vi "Init Panels.vi"(8 "error in (no error)":errorcluster, 11 "Editor in":refnum<class "Editor.lvclass">) -> (0 "error out":errorcluster, 3 "Editor out":refnum<class "Editor.lvclass">)   [LabVIEW 2020, in "VolatusGUIEditor.lvlib" / "Editor.lvclass"]
uses:
  Editor.lvclass
  Panels.ctl
  VolatusGUIControls/ElementEditorPanel/ElementEditorPanel.lvclass
  C:/dev/lv20CE/relink/lv-oopanel/OOPanel/Panel/Panel.lvclass
  ControlBindingPanel/ControlBindingPanel.lvclass
  Editor.lvclass/Editor.ctl
  lv-oopanel/OOPanel/Manager/Manager.lvclass
  Control List/Control List.lvclass
  VolatusGUIEditor.lvlib
  C:/dev/lv20CE/relink/volatus-gui-controls/VolatusGUIControls/ElementEditorPanel/ElementEditorPanel.lvclass
  C:/dev/lv20CE/relink/volatus-gui-controls/VolatusGUIEditor/ControlBindingPanel/ControlBindingPanel.lvclass
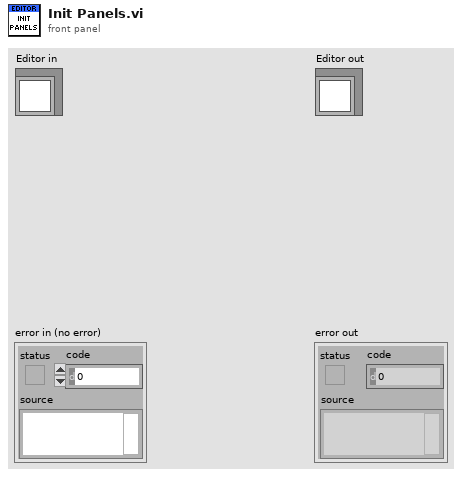
[diagram p1: front panel]
types:
  T1 = typedef "VolatusGUIEditor.lvlib/Editor.lvclass/Panels.ctl" = cluster{"Blank":refnum<class "ElementEditorPanel.lvclass">, "Binding":refnum<class "ControlBindingPanel.lvclass">}
  T2 = map{string, refnum<class "ElementEditorPanel.lvclass">}
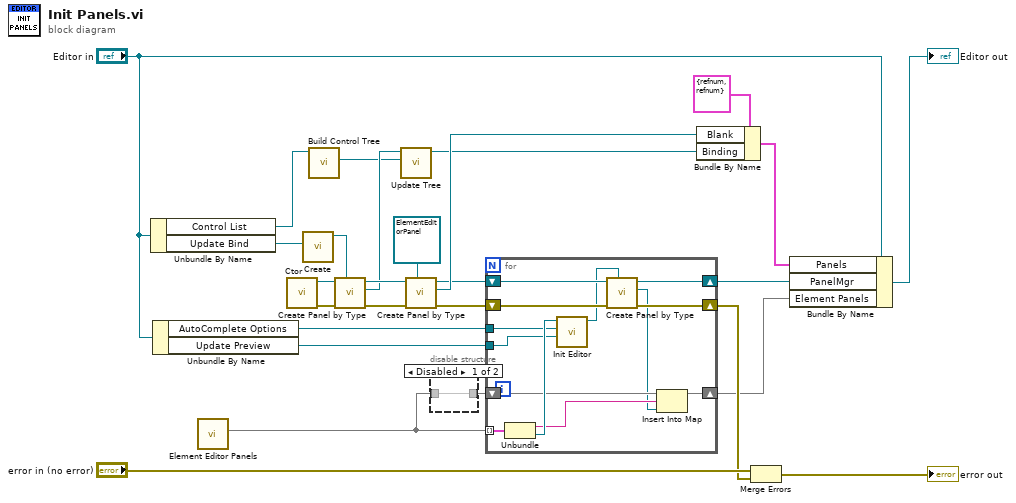
[diagram p0: block diagram]
diagram:
  n1 = Unbundle By Name("Editor in") -> ("Control List"=w12:refnum<class "Control List.lvclass">, "Update Bind"=w23:refnum<user-event>)
  n2 = Unbundle By Name("Editor in") -> ("AutoComplete Options"=w7:refnum<class "Shared Options.lvclass">, "Update Preview"=w3:refnum<user-event>)
  n3 = call "Element Editor Panels.vi"() -> ("Panels"=w5:T2)  [unwired: 11 in]
  n4 = call "Ctor.vi"() -> ("error out"=w25:errorcluster, "Manager out"=w26:refnum<class "Manager.lvclass">)  [unwired: 10 in]
  n5 = call "Create.vi"("Update Bind"=w23) -> ("ControlBindingPanel out"=w24:refnum<class "ControlBindingPanel.lvclass">)  [unwired: 9 in, 1 out]
  n6 = call "Build Control Tree.vi"("Control List in"=w12) -> ("Control Tree"=w11:refnum<class "Tree Map.lvclass">)  [unwired: 8 in, 2 out]
  n7 = call "Create Panel by Type.vi"("Panel Type"=w24, "error in (no error)"=w25, "Manager in"=w26) -> ("error out"=w18:errorcluster, "Panel"=w15:refnum<class "ControlBindingPanel.lvclass">, "Manager out"=w17:refnum<class "Manager.lvclass">)  [unwired: 6 in]
  n8 = call "Update Tree.vi"("Tree Map"=w11, "ControlBindingPanel in"=w15) -> ("ControlBindingPanel out"=w13:refnum<class "ControlBindingPanel.lvclass">)  [unwired: 8 in, 1 out]
  n9 = call "Create Panel by Type.vi"("Panel Type"=refnum<class "ElementEditorPanel.lvclass"> refnum ("VolatusGUIControls.lvlib:ElementEditorPanel.lvclass"), "error in (no error)"=w18, "Manager in"=w17) -> ("error out"=w8:errorcluster, "Panel"=w14:refnum<class "ElementEditorPanel.lvclass">, "Manager out"=w9:refnum<class "Manager.lvclass">)  [unwired: 6 in]
  n10 = disable-structure shown="Disabled" {
    disable-tunnel: [w28 _] -> w6
    disable-tunnel: w5 -> [w28 _]
    frame Disabled {
    }
    frame Enabled {
    }
  }
  n11 = for {
    shift-right: [w38] -> w4
    shift-left: w9 -> [w41]
    shift-right: [w37] -> w2
    shift-left: w8 -> [w40]
    tunnel: w5 -> [w39] mode=indexing
    tunnel: w7 -> [w35]
    shift-right: [w31] -> w1
    shift-left: w6 -> [w32]
    tunnel: w3 -> [w34]
    n12 = Unbundle(w39) -> (w30:string, "VolatusGUIControls.lvlib:ElementEditorPanel.lvclass"=w36:refnum<class "ElementEditorPanel.lvclass">)
    n13 = call "Init Editor.vi"("Update Preview"=w34, "Autocomplete Options"=w35, "ElementEditorPanel in"=w36) -> ("ElementEditorPanel out"=w33:refnum<class "ElementEditorPanel.lvclass">)  [unwired: 8 in]
    n14 = call "Create Panel by Type.vi"("Panel Type"=w33, "error in (no error)"=w40, "Manager in"=w41) -> ("error out"=w37:errorcluster, "Panel"=w29:refnum<class "ElementEditorPanel.lvclass">, "Manager out"=w38:refnum<class "Manager.lvclass">)  [unwired: 6 in]
    n15 = Insert Into Map(map in=w32, key=w30, value=w29) -> (map out=w31:T2)  [unwired: 2 out]
  }
  n16 = Bundle By Name(cluster=T1 {"Blank"=refnum, "Binding"=refnum} ("Panels"), "Blank"=w14, "Binding"=w13) -> (w20:T1)
  n17 = Merge Errors("error in (no error)", w2) -> (→"error out":errorcluster)
  n18 = Bundle By Name(cluster="Editor in", "Panels"=w20, "PanelMgr"=w4, "Element Panels"=w1) -> (→"Editor out":refnum<class "Editor.lvclass">)
